vi "Countdown 2.vi"() -> ()   [LabVIEW 2011]
panel:
  in  "stop":bool
  out "Boolean 7":bool
  out "Boolean 6":bool
  out "Boolean 5":bool
  out "Boolean 4":bool
  out "Boolean 3":bool
  out "Boolean 2":bool
  out "Boolean":bool
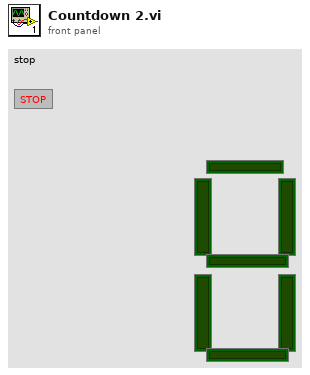
[diagram p1: front panel]
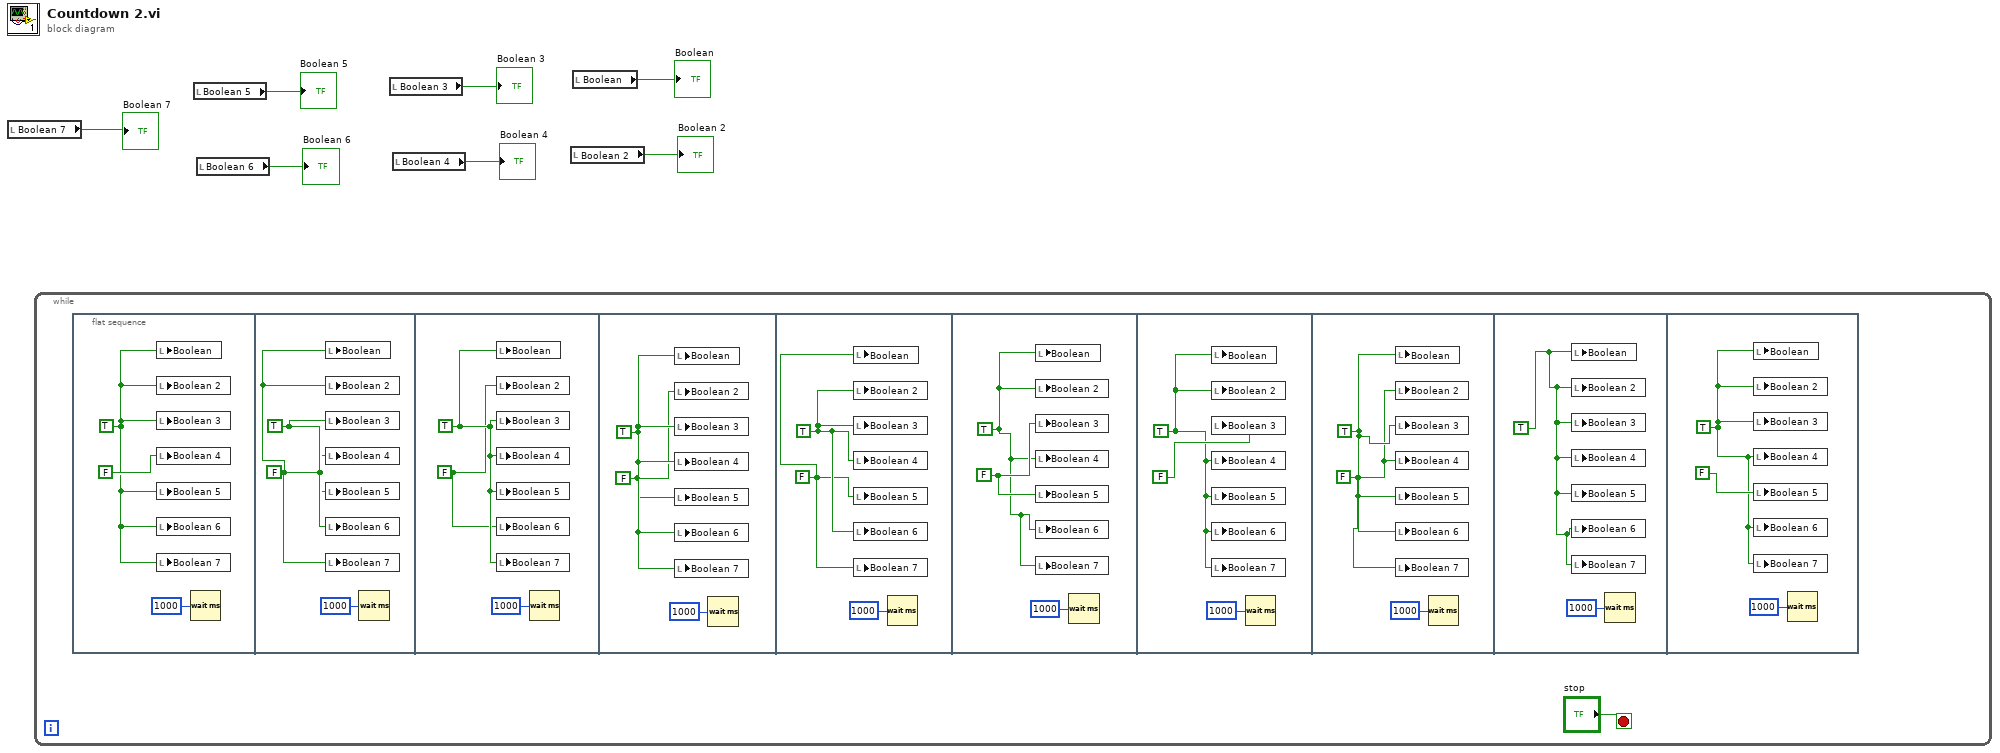
[diagram p0: block diagram]
diagram:
  n1 = local read "Boolean 7"() -> (→"Boolean 7":bool)
  n2 = while {
    stop <- "stop" stop-if-true
    n3 = flat-sequence {
      frame #0 {
        w9 = TRUE
        n4 = local write "Boolean"(w9) -> ()
        n5 = local write "Boolean 2"(w9) -> ()
        n6 = local write "Boolean 3"(w9) -> ()
        n7 = local write "Boolean 4"(FALSE) -> ()
        n8 = local write "Boolean 5"(w9) -> ()
        n9 = local write "Boolean 6"(w9) -> ()
        n10 = local write "Boolean 7"(w9) -> ()
        n11 = Wait (ms)(milliseconds to wait=u32 1000) -> ()  [unwired: 1 out]
      }
      frame #1 {
        w12 = FALSE
        w13 = TRUE
        n12 = local write "Boolean"(w12) -> ()
        n13 = local write "Boolean 2"(w12) -> ()
        n14 = local write "Boolean 3"(w13) -> ()
        n15 = local write "Boolean 4"(w12) -> ()
        n16 = local write "Boolean 5"(w12) -> ()
        n17 = local write "Boolean 6"(w13) -> ()
        n18 = local write "Boolean 7"(w12) -> ()
        n19 = Wait (ms)(milliseconds to wait=u32 1000) -> ()  [unwired: 1 out]
      }
      frame #2 {
        w15 = FALSE
        w16 = TRUE
        n20 = local write "Boolean"(w16) -> ()
        n21 = local write "Boolean 2"(w15) -> ()
        n22 = local write "Boolean 3"(w16) -> ()
        n23 = local write "Boolean 4"(w16) -> ()
        n24 = local write "Boolean 5"(w16) -> ()
        n25 = local write "Boolean 6"(w15) -> ()
        n26 = local write "Boolean 7"(w16) -> ()
        n27 = Wait (ms)(milliseconds to wait=u32 1000) -> ()  [unwired: 1 out]
      }
      frame #3 {
        w18 = FALSE
        w19 = TRUE
        n28 = local write "Boolean"(w19) -> ()
        n29 = local write "Boolean 2"(w18) -> ()
        n30 = local write "Boolean 3"(w19) -> ()
        n31 = local write "Boolean 4"(w19) -> ()
        n32 = local write "Boolean 5"(w18) -> ()
        n33 = local write "Boolean 6"(w19) -> ()
        n34 = local write "Boolean 7"(w19) -> ()
        n35 = Wait (ms)(milliseconds to wait=u32 1000) -> ()  [unwired: 1 out]
      }
      frame #4 {
        w21 = FALSE
        w22 = TRUE
        n36 = local write "Boolean"(w21) -> ()
        n37 = local write "Boolean 2"(w22) -> ()
        n38 = local write "Boolean 3"(w22) -> ()
        n39 = local write "Boolean 4"(w22) -> ()
        n40 = local write "Boolean 5"(w21) -> ()
        n41 = local write "Boolean 6"(w22) -> ()
        n42 = local write "Boolean 7"(w21) -> ()
        n43 = Wait (ms)(milliseconds to wait=u32 1000) -> ()  [unwired: 1 out]
      }
      frame #5 {
        w25 = FALSE
        w24 = TRUE
        n44 = local write "Boolean"(w24) -> ()
        n45 = local write "Boolean 2"(w24) -> ()
        n46 = local write "Boolean 3"(w25) -> ()
        n47 = local write "Boolean 4"(w24) -> ()
        n48 = local write "Boolean 5"(w25) -> ()
        n49 = local write "Boolean 6"(w24) -> ()
        n50 = local write "Boolean 7"(w24) -> ()
        n51 = Wait (ms)(milliseconds to wait=u32 1000) -> ()  [unwired: 1 out]
      }
      frame #6 {
        w27 = TRUE
        n52 = local write "Boolean"(w27) -> ()
        n53 = local write "Boolean 2"(w27) -> ()
        n54 = local write "Boolean 3"(FALSE) -> ()
        n55 = local write "Boolean 4"(w27) -> ()
        n56 = local write "Boolean 5"(w27) -> ()
        n57 = local write "Boolean 6"(w27) -> ()
        n58 = local write "Boolean 7"(w27) -> ()
        n59 = Wait (ms)(milliseconds to wait=u32 1000) -> ()  [unwired: 1 out]
      }
      frame #7 {
        w30 = FALSE
        w31 = TRUE
        n60 = local write "Boolean"(w31) -> ()
        n61 = local write "Boolean 2"(w30) -> ()
        n62 = local write "Boolean 3"(w31) -> ()
        n63 = local write "Boolean 4"(w30) -> ()
        n64 = local write "Boolean 5"(w30) -> ()
        n65 = local write "Boolean 6"(w31) -> ()
        n66 = local write "Boolean 7"(w30) -> ()
        n67 = Wait (ms)(milliseconds to wait=u32 1000) -> ()  [unwired: 1 out]
      }
      frame #8 {
        w33 = TRUE
        n68 = local write "Boolean"(w33) -> ()
        n69 = local write "Boolean 2"(w33) -> ()
        n70 = local write "Boolean 3"(w33) -> ()
        n71 = local write "Boolean 4"(w33) -> ()
        n72 = local write "Boolean 5"(w33) -> ()
        n73 = local write "Boolean 6"(w33) -> ()
        n74 = local write "Boolean 7"(w33) -> ()
        n75 = Wait (ms)(milliseconds to wait=u32 1000) -> ()  [unwired: 1 out]
      }
      frame #9 {
        w35 = TRUE
        n76 = local write "Boolean"(w35) -> ()
        n77 = local write "Boolean 2"(w35) -> ()
        n78 = local write "Boolean 3"(w35) -> ()
        n79 = local write "Boolean 4"(w35) -> ()
        n80 = local write "Boolean 5"(FALSE) -> ()
        n81 = local write "Boolean 6"(w35) -> ()
        n82 = local write "Boolean 7"(w35) -> ()
        n83 = Wait (ms)(milliseconds to wait=u32 1000) -> ()  [unwired: 1 out]
      }
    }
  }
  n84 = local read "Boolean 5"() -> (→"Boolean 5":bool)
  n85 = local read "Boolean 6"() -> (→"Boolean 6":bool)
  n86 = local read "Boolean 3"() -> (→"Boolean 3":bool)
  n87 = local read "Boolean 4"() -> (→"Boolean 4":bool)
  n88 = local read "Boolean 2"() -> (→"Boolean 2":bool)
  n89 = local read "Boolean"() -> (→"Boolean":bool)
